vi "Read Power.vi"(8 "error in (no error)":errorcluster, 11 "SimpleDevice in":refnum<class "SimpleDevice.lvclass">) -> (0 "error out":errorcluster, 2 "Power":bool, 3 "SimpleDevice out":refnum<class "SimpleDevice.lvclass">)   [LabVIEW 2021, in "SimpleDevice.lvlib" / "SimpleDevice.lvclass"]
uses:
  SimpleDevice.lvclass
  SimpleDevice.lvclass/SimpleDevice.ctl
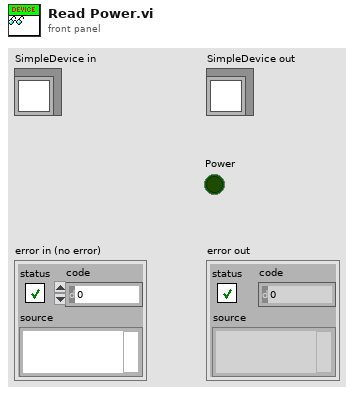
[diagram p1: front panel]
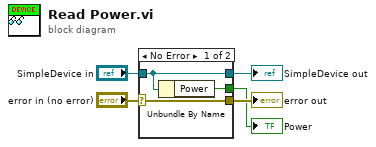
[diagram p0: block diagram]
diagram:
  n1 = case shown="No Error" "error in (no error)" {
    selector: "error in (no error)" -> [w8 w9]
    tunnel: [w8 w9] -> w4
    tunnel: [w7 w10] -> w2
    tunnel: "SimpleDevice in" -> [w7 w10]
    tunnel: [w6 _] -> w1
    frame No Error {
      n2 = Unbundle By Name(w7) -> ("Power"=w6:bool)
    }
    frame Error {
    }
  }
  "error out" <- w4
  "SimpleDevice out" <- w2
  "Power" <- w1
